vi "From Serial Form.vi"(6 "Serial Version":T1, 10 "Deserializer in":refnum<class "Deserializer.lvclass">, 11 "CRDS Cell Data in":refnum<class "CRDS Cell Data.lvclass">) -> (0 "error out":errorcluster, 2 "Deserializer out":refnum<class "Deserializer.lvclass">, 3 "CRDS Cell Data out":refnum<class "CRDS Cell Data.lvclass">)   [LabVIEW 2014, in "CRDS Cell Data.lvclass"]
uses:
  CRDS Cell Data.lvclass
  <vilib>/NI/AQ Character Lineator/Serializable/Serializable.lvclass
  <vilib>/NI/AQ Character Lineator/Serializable/Remove Single.vi
  <vilib>/NI/AQ Character Lineator/Serializable/Remove Single Array.vi
  <vilib>/NI/AQ Character Lineator/Serializable/Remove Int16 Array.vi
  Data/Data.lvclass
  <vilib>/NI/AQ Character Lineator/Serialization Common/Serial Version.ctl
  <vilib>/NI/AQ Character Lineator/Serialization Common/Serialization Common.lvlib
  <vilib>/NI/AQ Character Lineator/Deserializer/Deserializer.lvclass
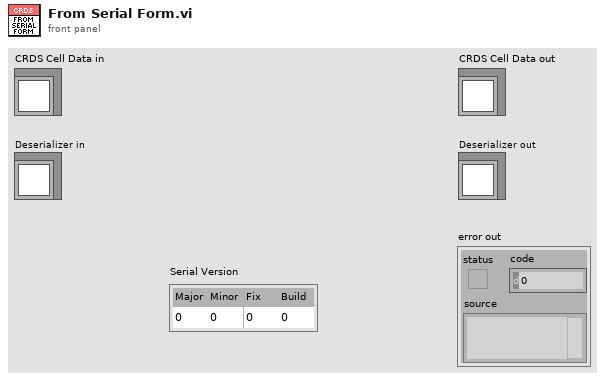
[diagram p1: front panel]
types:
  T1 = typedef "Serialization Common.lvlib/Serial Version.ctl" = cluster{"Major":u16, "Minor":u16, "Fix":u16, "Build":u16}
  T2 = cluster{"[0]":sgl, "[1]":sgl, "[2]":sgl, "[3]":sgl, "[4]":sgl, "[5]":sgl, "[6]":sgl, "[7]":sgl, "[8]":sgl}
  T3 = cluster{"[0]":sgl, "[1]":sgl, "[2]":sgl, "[3]":sgl, "[4]":sgl, "[5]":sgl, "[6]":sgl}
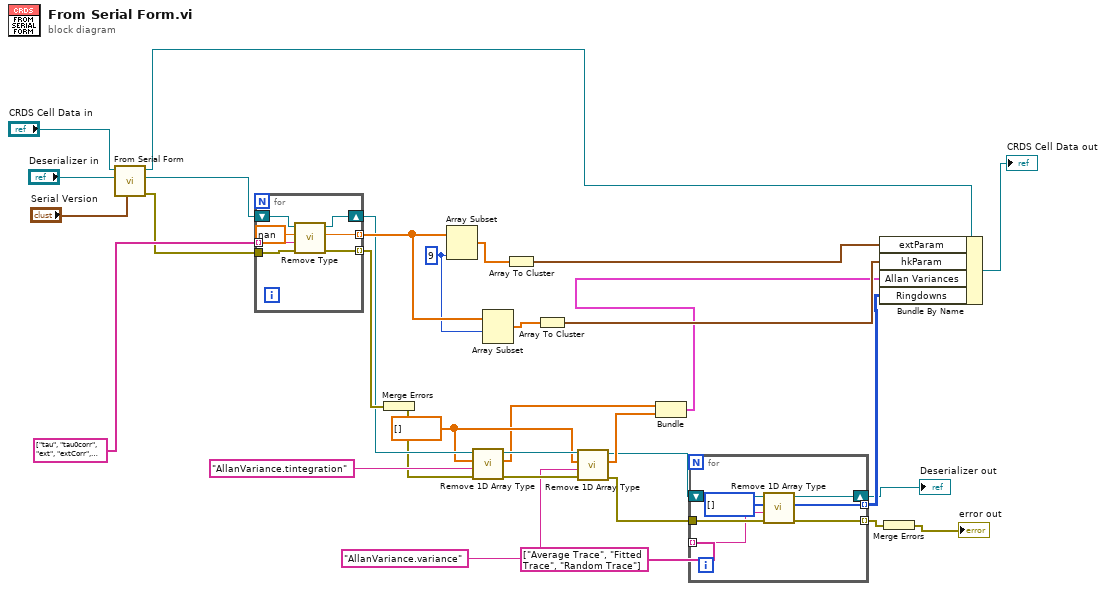
[diagram p0: block diagram]
diagram:
  w12 = sgl[] [] ("Default Value")
  w24 = 9 ("length")
  n1 = call-parent "From Serial Form.vi"("Serial Version"="Serial Version", "Deserializer in"="Deserializer in", "Data in"="CRDS Cell Data in") -> ("error out"=w27:errorcluster, "Deserializer out"=w28:refnum<class "Deserializer.lvclass">, "Data out"=w26:refnum<class "CRDS Cell Data.lvclass">)  [unwired: 6 in]
  n2 = for {
    tunnel: string[] ["tau", "tau0corr", "ext", "extCorr", "stdevTau", "etau", "taucorr", "tau0", "max", "rhdilfac", "Q", "Tmean", "extdilfac", "rhcell", "P", "T"] -> [w39] mode=indexing
    shift-right: [w36] -> w16
    shift-left: w28 -> [w37]
    tunnel: w27 -> [w35]
    tunnel: [w34] -> w25 mode=indexing
    tunnel: [w33] -> w18 mode=indexing
    n3 = call-poly <vilib>:"Remove Type.vi"("error in (no error)"=w35, "Name"=w39, "Default Value"=sgl nan, "Deserializer in"=w37) -> ("error out"=w33:errorcluster, "Numeric"=w34:sgl, "Deserializer out"=w36:refnum<class "Deserializer.lvclass">)  [unwired: 4 in, 1 out]
  }
  n4 = Merge Errors(w18) -> (w3:errorcluster)
  n5 = Array Subset(array=w25, length=w24) -> (w23:sgl[])  [unwired: 1 in]
  n6 = call-poly <vilib>:"Remove 1D Array Type.vi"("error in (no error)"=w3, "Name"="AllanVariance.tintegration", "Default Value"=w12, "Deserializer in"=w16) -> ("error out"=w14:errorcluster, "Singles"=w10:sgl[], "Deserializer out"=w15:refnum<class "Deserializer.lvclass">)  [unwired: 4 in, 1 out]
  n7 = Array Subset(array=w25, index=w24) -> (w21:sgl[])  [unwired: 1 in]
  n8 = Array To Cluster(array=w23) -> (cluster=w22:T2)
  n9 = Array To Cluster(array=w21) -> (cluster=w20:T3)
  n10 = call-poly <vilib>:"Remove 1D Array Type.vi"("error in (no error)"=w14, "Name"="AllanVariance.variance", "Default Value"=w12, "Deserializer in"=w15) -> ("error out"=w7:errorcluster, "Singles"=w11:sgl[], "Deserializer out"=w8:refnum<class "Deserializer.lvclass">)  [unwired: 4 in, 1 out]
  n11 = Bundle("Singles"=w10, "Singles"=w11) -> (w9:cluster{"Singles":sgl[], "Singles":sgl[]})  [unwired: 1 in]
  n12 = for {
    shift-right: [w45] -> w4
    shift-left: w8 -> [w46]
    tunnel: [w44] -> w2 mode=indexing
    tunnel: w7 -> [w43]
    tunnel: string[] ["Average Trace", "Fitted Trace", "Random Trace"] -> [w42] mode=indexing
    tunnel: [w40] -> w5 mode=indexing
    n13 = call-poly <vilib>:"Remove 1D Array Type.vi"("error in (no error)"=w43, "Name"=w42, "Default Value"=i16[] [], "Deserializer in"=w46) -> ("error out"=w44:errorcluster, "Integers"=w40:i16[], "Deserializer out"=w45:refnum<class "Deserializer.lvclass">)  [unwired: 4 in, 1 out]
  }
  "Deserializer out" <- w4
  n14 = Bundle By Name(cluster=w26, "extParam"=w22, "hkParam"=w20, "Allan Variances"=w9, "Ringdowns"=w5) -> (→"CRDS Cell Data out":refnum<class "CRDS Cell Data.lvclass">)
  n15 = Merge Errors(w2) -> (→"error out":errorcluster)
